vi "AddToVariantAttributes.vi"(8 "ErrorIn":errorcluster, 9 "DataInIn":variant, 10 "PersistentData":variant, 11 "Object":refnum<class>) -> (0 "ErrorOut":errorcluster, 1 "DataInOut":variant)   [LabVIEW 2021]
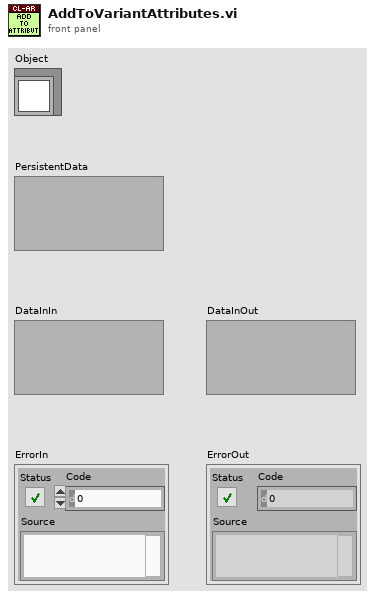
[diagram p1: front panel]
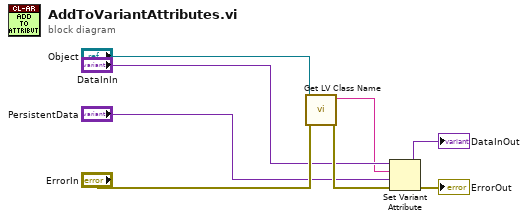
[diagram p0: block diagram]
diagram:
  n1 = call <vilib>:"Get LV Class Name.vi"("error in (no error)"="ErrorIn", "object"="Object") -> ("error out"=w6:errorcluster, "class name"=w2:string)  [unwired: 8 in]
  n2 = Set Variant Attribute(Variant="DataInIn", name=w2, value="PersistentData", error in=w6) -> (Variant out=→"DataInOut":variant, error out=→"ErrorOut":errorcluster)  [unwired: 1 out]
